vi "DAQ (SubVI).vi"(8 "error in (no error)":errorcluster, 11 "output cluster":T2) -> (0 "error out":errorcluster)   [LabVIEW 2016]
uses:
  Que Cluster TD.ctl
  Que Attributes TD.ctl
  Que enum td.ctl
  External data TD.ctl
  <vilib>/DAQmx/read.llb/DAQmx Read (Analog 2D DBL NChan NSamp).vi
  <vilib>/DAQmx/create/channels.llb/DAQmx Create Channel (AI-Voltage-Basic).vi
  <vilib>/DAQmx/configure/timing.llb/DAQmx Timing (Sample Clock).vi
  <vilib>/DAQmx/miscellaneous.llb/DAQmx Fill In Error Info.vi
panel:
  in  "rate":dbl=1000.0 format="%#_13g"
  in  "samples per channel":i32=100
  out "Waveform Graph 3":dbl[](graph)
  out "Waveform Graph 2":dbl[](graph)
  out "External Data":dbl[](graph)
  in  "External Data TD":T1
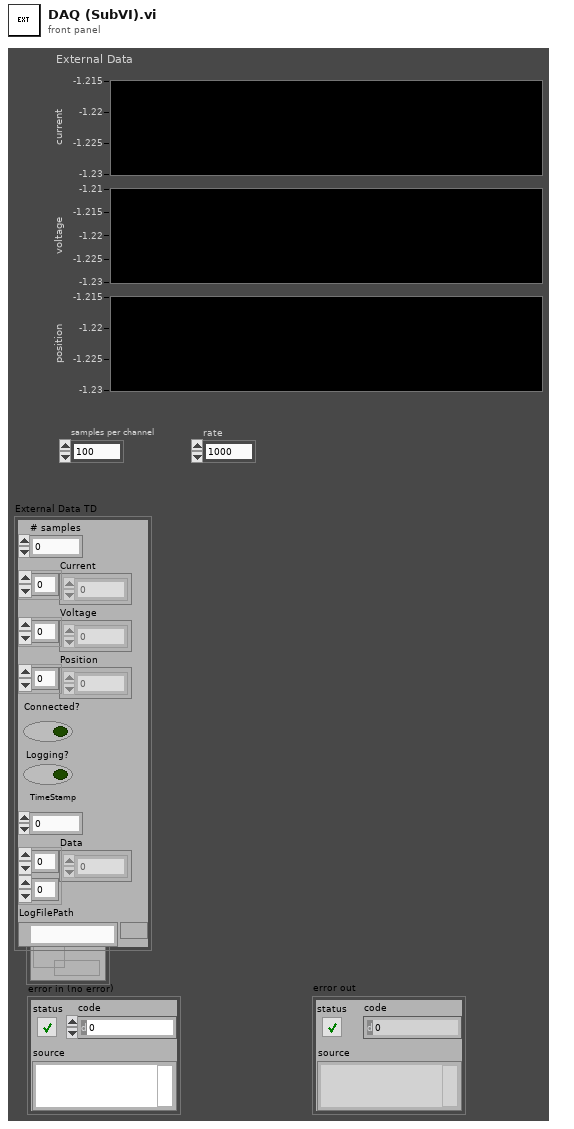
[diagram p1: front panel]
types:
  T1 = typedef "External data TD.ctl" = cluster{"# samples":i32, "Current":dbl[], "Voltage":dbl[], "Position":dbl[], "Connected?":bool, "Logging?":bool, "TimeStamp":dbl, "Data":dbl[][], "LogFilePath":path}
  T2 = typedef "Que Cluster TD.ctl" = cluster{"Main":refnum<queue>, "ZMQ_SUB":refnum<queue>, "External":refnum<queue>, "Vibration":refnum<queue>, "ZMQ_REQ":refnum<queue>}
  T3 = typedef "Que Attributes TD.ctl" = cluster{"Que States":T4, "String":string, "Boolean":bool, "Double":dbl, "U16":u16}
  T4 = typedef "Que enum td.ctl" = enum16{"Stop", "Start", "Update D_HW", "Initialize", "Exit", "Read", "Write", "Plot", "Log", "Stop Log", "Start Log", "Wait"}
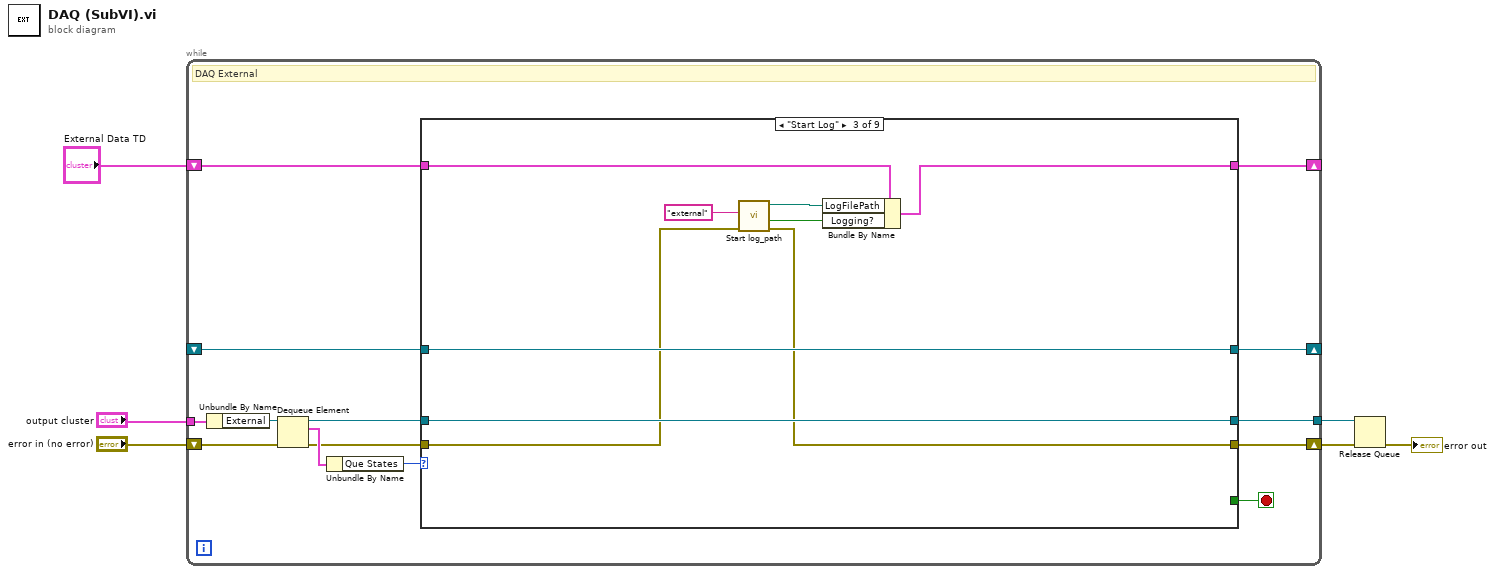
[diagram p0: block diagram]
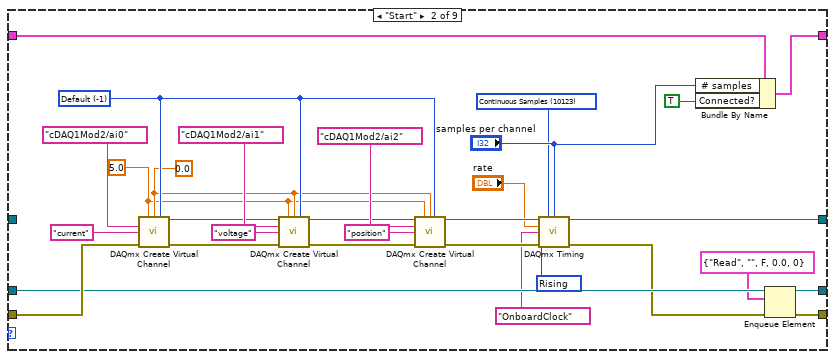
[diagram p3: hidden frame]
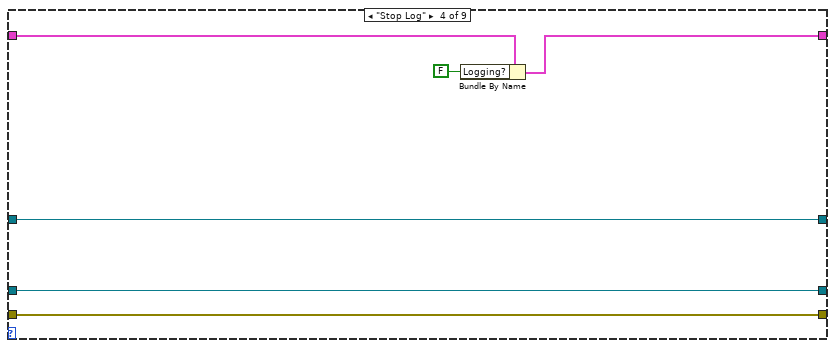
[diagram p4: hidden frame]
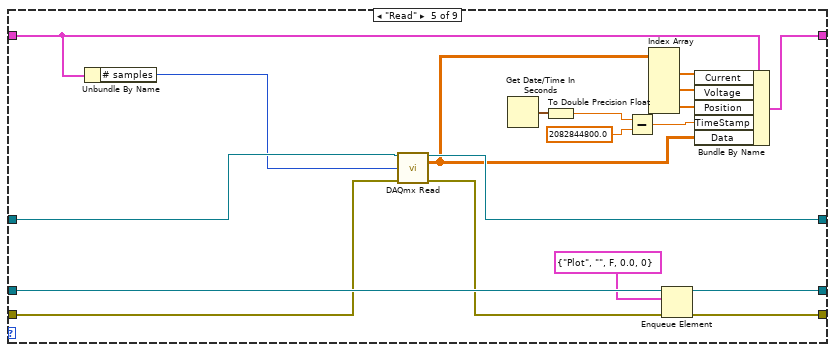
[diagram p5: hidden frame]
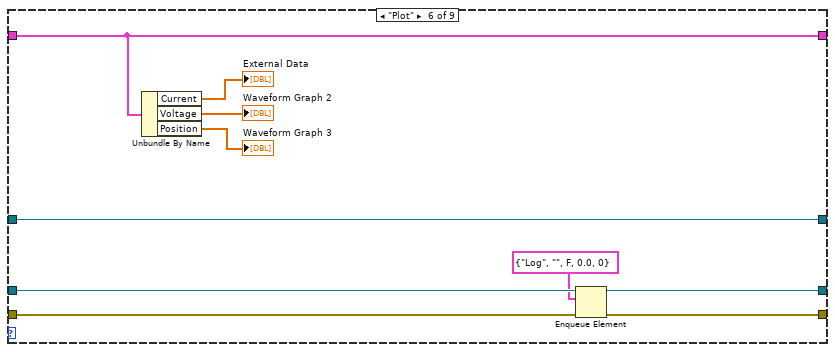
[diagram p6: hidden frame]
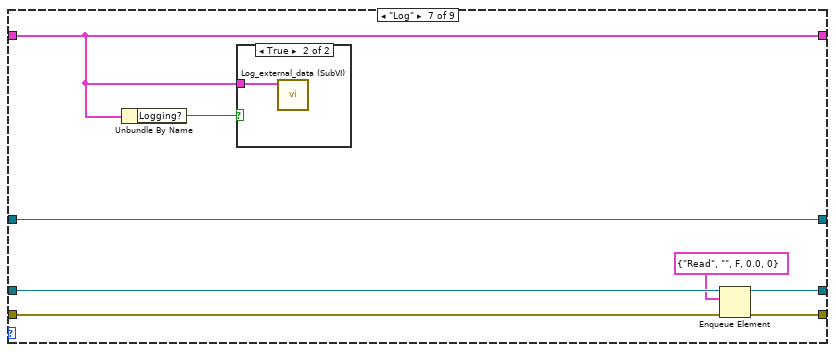
[diagram p7: hidden frame]
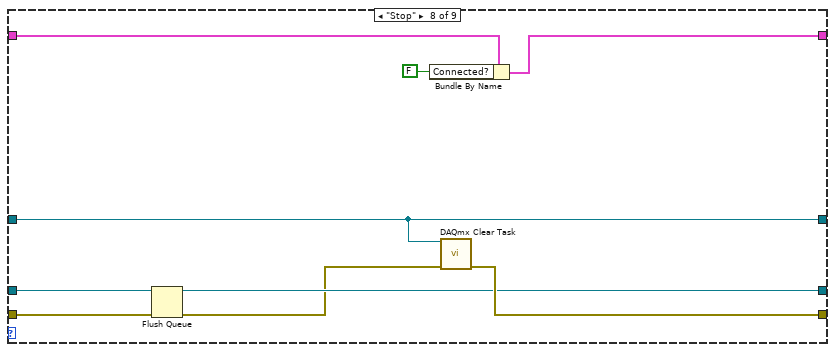
[diagram p9: hidden frame]
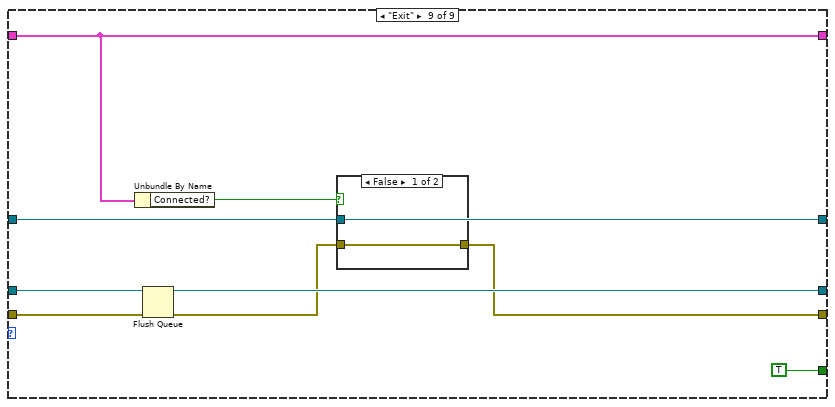
[diagram p10: hidden frame]
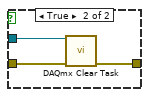
[diagram p11: hidden frame]
diagram:
  n1 = while {
    tunnel: "output cluster" -> [w20]
    tunnel: [w14] -> w5
    shift-right: [w13] -> w6
    shift-left: "error in (no error)" -> [w18]
    shift-right: [w10] -> _
    shift-left: _ -> [w9]
    shift-right: [w7] -> _
    shift-left: "External Data TD" -> [w8]
    stop <- w11 stop-if-true
    # "DAQ External"
    n2 = Unbundle By Name(w20) -> ("External"=w19:refnum<queue>)
    n3 = Dequeue Element(queue=w19, error in (no error)=w18) -> (queue out=w15:refnum<queue>, element=w17:T3, error out=w16:errorcluster)  [unwired: 1 in, 1 out]
    n4 = Unbundle By Name(w17) -> ("Que States"=w12:T4)
    n5 = case shown="\"Start Log\"" w12 {
      tunnel: w16 -> [w21 w54 w58 w64 w84 w91 w102 w112 w119]
      tunnel: w15 -> [w22 w41 w63 w69 w87 w93 w104 w111 w121]
      tunnel: [w22 w40 w63 w69 w86 w92 w103 w110 w120] -> w14
      tunnel: [w21 w42 w57 w64 w88 w90 w101 w113 w117] -> w13
      tunnel: [_ _ _ _ _ _ _ _ TRUE] -> w11
      tunnel: [w24 w30 w62 w68 w82 w98 w106 w108 w124] -> w10
      tunnel: w9 -> [w24 _ w62 w68 w73 w98 w106 w108 w124]
      tunnel: w8 -> [w23 w34 w61 w67 w72 w97 w99 w116 w123]
      tunnel: [w23 w33 w60 w66 w81 w97 w99 w115 w123] -> w7
      frame "Initialize", Default {
      }
      frame "Start" {
        w25 = 10280 items=["Rising"=10280, "Falling"=10171] ("active edge")
        w26 = 10123 items=["Finite Samples"=10178, "Continuous Samples"=10123, "Hardware Timed Single Point"=12522] ("sample mode")
        w47 = 0.0 ("minimum value")
        w46 = 5.0 ("maximum value")
        w50 = -1 items=["Default"=-1, "RSE"=10083, "NRSE"=10078, "Differential"=10106, "Pseudodifferential"=12529] ("input terminal configuration")
        n6 = call-poly <vilib>:"DAQmx Create Virtual Channel.vi"("maximum value"=w46, "minimum value"=w47, "input terminal configuration"=w50, "physical channels"=tag "cDAQ1Mod2/ai0", "name to assign"="current", "error in"=w54) -> ("task out"=w38:refnum<k21>, "error out"=w52:errorcluster)  [unwired: 8 in]
        n7 = call-poly <vilib>:"DAQmx Create Virtual Channel.vi"("task in"=w38, "maximum value"=w46, "minimum value"=w47, "input terminal configuration"=w50, "physical channels"=tag "cDAQ1Mod2/ai1", "name to assign"="voltage", "error in"=w52) -> ("task out"=w37:refnum<k21>, "error out"=w51:errorcluster)  [unwired: 7 in]
        n8 = call-poly <vilib>:"DAQmx Create Virtual Channel.vi"("task in"=w37, "maximum value"=w46, "minimum value"=w47, "input terminal configuration"=w50, "physical channels"=tag "cDAQ1Mod2/ai2", "name to assign"="position", "error in"=w51) -> ("task out"=w36:refnum<k21>, "error out"=w35:errorcluster)  [unwired: 7 in]
        n9 = call-poly <vilib>:"DAQmx Timing.vi"("task/channels in"=w36, "sample mode"=w26, "samples per channel"="samples per channel", "rate"="rate", "source"=tag "OnboardClock", "active edge"=w25, "error in"=w35) -> ("task out"=w30:refnum<k21>, "error out"=w29:errorcluster)  [unwired: 7 in]
        n10 = Bundle By Name(cluster=w34, "# samples"="samples per channel", "Connected?"=TRUE) -> (w33:T1)
        n11 = Enqueue Element(queue=w41, element=T3 {"Que States"=enum."Read", "String"="", "Boolean"=FALSE, "Double"=0.0, "U16"=0}, error in (no error)=w29) -> (queue out=w40:refnum<queue>, error out=w42:errorcluster)  [unwired: 1 in, 1 out]
      }
      frame "Start Log" {
        n12 = call "Start log_path.vi"("error in (no error)"=w58, "Data type"="external") -> ("error out"=w57:errorcluster, "Logging"=w59:bool, "Path"=w55:path)  [unwired: 7 in]
        n13 = Bundle By Name(cluster=w61, "LogFilePath"=w55, "Logging?"=w59) -> (w60:T1)
      }
      frame "Stop Log" {
        n14 = Bundle By Name(cluster=w67, "Logging?"=FALSE) -> (w66:T1)
      }
      frame "Read" {
        n15 = Unbundle By Name(w72) -> ("# samples"=w71:i32)
        n16 = call-poly <vilib>:"DAQmx Read.vi"("task/channels in"=w73, "number of samples per channel"=w71, "error in"=w84) -> ("task out"=w82:refnum<k21>, "data"=w70:dbl[][], "error out"=w83:errorcluster)  [unwired: 10 in]
        n17 = Get Date/Time In Seconds() -> (seconds since 1Jan1904=w77:timestamp)
        n18 = To Double Precision Float(number=w77) -> (double precision float=w76:dbl)
        n19 = Subtract(x=w76, y=2082844800.0 ("Epoch Delta (s)")) -> (x-y=w74:dbl)
        n20 = Index Array(array=w70) -> (element #1=w80:dbl[], element #2=w79:dbl[], element #3=w78:dbl[])  [unwired: 6 in]
        n21 = Enqueue Element(queue=w87, element=T3 {"Que States"=enum."Plot", "String"="", "Boolean"=FALSE, "Double"=0.0, "U16"=0}, error in (no error)=w83) -> (queue out=w86:refnum<queue>, error out=w88:errorcluster)  [unwired: 1 in, 1 out]
        n22 = Bundle By Name(cluster=w72, "Current"=w80, "Voltage"=w79, "Position"=w78, "TimeStamp"=w74, "Data"=w70) -> (w81:T1)
      }
      frame "Plot" {
        n23 = Unbundle By Name(w97) -> ("Current"=→"External Data":dbl[], "Voltage"=→"Waveform Graph 2":dbl[], "Position"=→"Waveform Graph 3":dbl[])
        n24 = Enqueue Element(queue=w93, element=T3 {"Que States"=enum."Log", "String"="", "Boolean"=FALSE, "Double"=0.0, "U16"=0}, error in (no error)=w91) -> (queue out=w92:refnum<queue>, error out=w90:errorcluster)  [unwired: 1 in, 1 out]
      }
      frame "Log" {
        n25 = Unbundle By Name(w99) -> ("Logging?"=w105:bool)
        n26 = case shown="True" w105 {
          tunnel: w99 -> [_ w107]
          frame False {
          }
          frame True {
            n27 = call "Log_external_data (SubVI).vi"("External Data TD"=w107) -> ()  [unwired: 11 in]
          }
        }
        n28 = Enqueue Element(queue=w104, element=T3 {"Que States"=enum."Read", "String"="", "Boolean"=FALSE, "Double"=0.0, "U16"=0}, error in (no error)=w102) -> (queue out=w103:refnum<queue>, error out=w101:errorcluster)  [unwired: 1 in, 1 out]
      }
      frame "Stop" {
        n29 = Flush Queue(queue=w111, error in (no error)=w112) -> (queue out=w110:refnum<queue>, error out=w109:errorcluster)  [unwired: 1 out]
        n30 = Bundle By Name(cluster=w116, "Connected?"=FALSE) -> (w115:T1)
        n31 = call <vilib>:"DAQmx Clear Task.vi"("task in"=w108, "error in"=w109) -> ("error out"=w113:errorcluster)  [unwired: 13 in]
      }
      frame "Exit" {
        n32 = Unbundle By Name(w123) -> ("Connected?"=w122:bool)
        n33 = Flush Queue(queue=w121, error in (no error)=w119) -> (queue out=w120:refnum<queue>, error out=w118:errorcluster)  [unwired: 1 out]
        n34 = case shown="False" w122 {
          tunnel: w124 -> [_ w129]
          tunnel: w118 -> [w126 w128]
          tunnel: [w126 w127] -> w117
          frame False {
          }
          frame True {
            n35 = call <vilib>:"DAQmx Clear Task.vi"("task in"=w129, "error in"=w128) -> ("error out"=w127:errorcluster)  [unwired: 13 in]
          }
        }
      }
    }
  }
  n36 = Release Queue(queue=w5, error in (no error)=w6) -> (error out=→"error out":errorcluster)  [unwired: 1 in, 2 out]
